vi "saveDelayConfig_烧录.vi"() -> (2 "读取":dbl, 3 "Q写入":dbl, 5 "S写入":dbl)   [LabVIEW 2011]
uses:
  <vilib>/Utility/file.llb/Write To Spreadsheet File (string).vi
  <vilib>/Utility/file.llb/Read From Spreadsheet File (string).vi
panel:
  in  "SFP+写入延时（单位：ms）":dbl
  out "DelayConfigFile":path caption="路径副本"
  in  "保存按钮":bool
  in  "读取延时（单位：ms）":dbl
  in  "QSFP+写入延时（单位：ms）":dbl
  # "建议值：200，可根据实际情况进行调整"
  # "建议值：100，可根据实际情况进行调整"
  # "建议值：100，可根据实际情况进行调整"
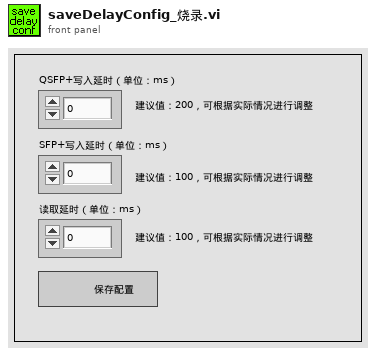
[diagram p1: front panel]
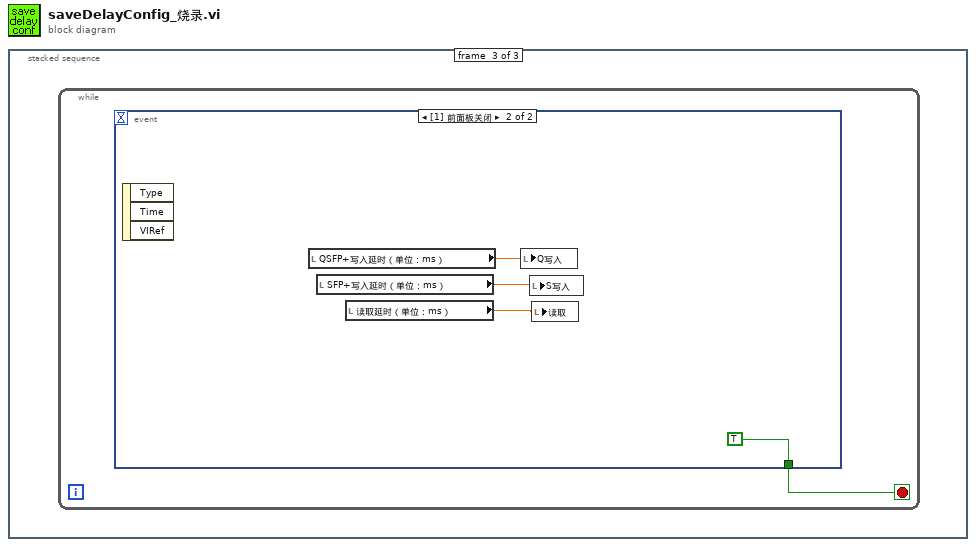
[diagram p0: block diagram]
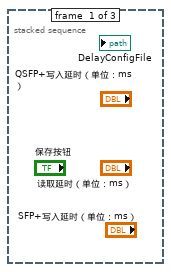
[diagram p2: hidden frame]
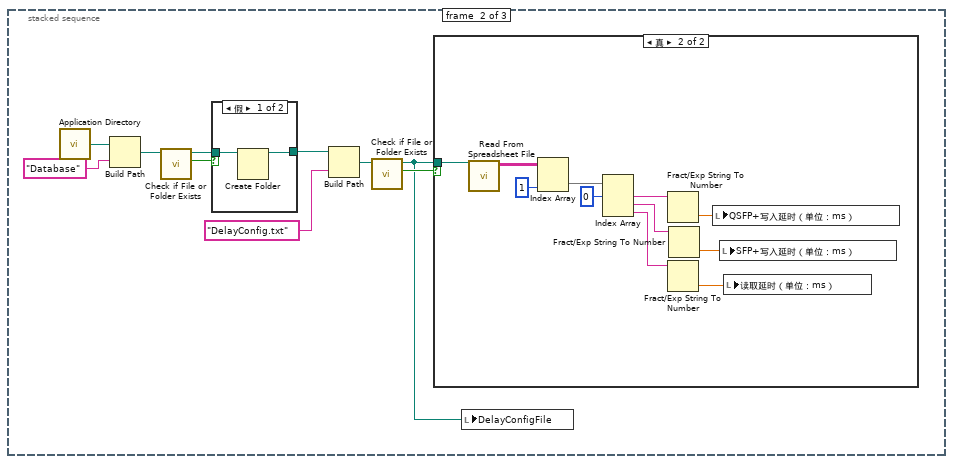
[diagram p3: hidden frame]
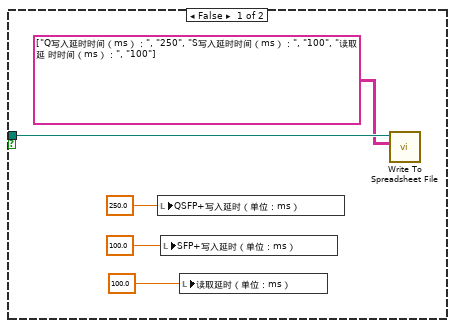
[diagram p4: hidden frame]
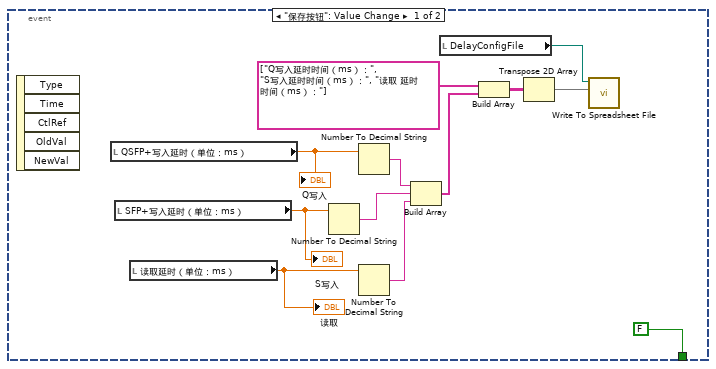
[diagram p6: hidden frame]
diagram:
  n1 = stacked-sequence {
    frame #0 {
    }
    frame #1 {
      n2 = call <vilib>:"Application Directory.vi"() -> ("Application Directory"=w10:path)
      n3 = Build Path(base path=w10, name or relative path="Database" ("名称或相对路径")) -> (appended path=w8:path)
      n4 = call <vilib>:"Check if File or Folder Exists.vi"("path"=w8) -> ("file or folder exists?"=w7:bool, "dup path"=w6:path)  [unwired: 8 in, 1 out]
      n5 = case shown="假" w7 {
        tunnel: w6 -> [w28 w29]
        tunnel: [w27 w29] -> w5
        frame False {
          n6 = Create Folder(path (use dialog)=w28) -> (created path=w27:path)  [unwired: 2 in, 2 out]
        }
        frame True {
        }
      }
      n7 = Build Path(base path=w5, name or relative path="DelayConfig.txt" ("名称或相对路径")) -> (appended path=w3:path)
      n8 = call <vilib>:"Check if File or Folder Exists.vi"("path"=w3) -> ("file or folder exists?"=w2:bool, "dup path"=w1:path)  [unwired: 8 in, 1 out]
      n9 = case shown="真" w2 {
        tunnel: w1 -> [w15 w26]
        frame False {
          n10 = local write "QSFP+写入延时（单位：ms）"(250.0 ("写入延时（单位：ms）")) -> ()
          n11 = local write "SFP+写入延时（单位：ms）"(100.0 ("SFP+写入延时（单位：ms）")) -> ()
          n12 = local write "读取延时（单位：ms）"(100.0 ("读取延时（单位：ms）")) -> ()
          n13 = call-poly <vilib>:"Write To Spreadsheet File.vi"("2D data"=string[][] [["Q写入延时时间（ms）：", "250"], ["S写入延时时间（ms）：", "100"], ["读取 延 时时间（ms）：", "100"]], "file path (dialog if empty)"=w15) -> ()  [unwired: 6 in, 1 out]
        }
        frame True {
          n14 = call-poly <vilib>:"Read From Spreadsheet File.vi"("file path (dialog if empty)"=w26) -> ("all rows"=w25:string[][])  [unwired: 6 in, 4 out]
          n15 = Index Array(array=w25, index (col)=1 ("禁用的索引 (列)")) -> (element=w23:string[])  [unwired: 1 in]
          n16 = Index Array(array=w23, index #1=0 ("索引")) -> (element #1=w21:string, element #2=w16:string, element #3=w18:string)  [unwired: 2 in]
          n17 = Fract/Exp String To Number(string=w21) -> (number=w20:dbl)  [unwired: 3 in, 1 out]
          n18 = Fract/Exp String To Number(string=w18) -> (number=w19:dbl)  [unwired: 3 in, 1 out]
          n19 = Fract/Exp String To Number(string=w16) -> (number=w17:dbl)  [unwired: 3 in, 1 out]
          n20 = local write "QSFP+写入延时（单位：ms）"(w20) -> ()
          n21 = local write "SFP+写入延时（单位：ms）"(w17) -> ()
          n22 = local write "读取延时（单位：ms）"(w19) -> ()
        }
      }
      n23 = local write "DelayConfigFile"(w1) -> ()
    }
    frame #2 {
      n24 = while {
        stop <- w30 stop-if-true
        n25 = event shown="[1] 前面板关闭" {
          selector: _ -> [_ _]
          dyn-events: _ -> [_ _]
          timeout: _ -> [_ _]
          tunnel: [FALSE TRUE] -> w30
          event "保存按钮": Value Change {
            n26 = event-data() -> ()  [unwired: 1 in, 5 out]
            n27 = local read "QSFP+写入延时（单位：ms）"() -> (w42:dbl)
            "Q写入" <- w42
            n28 = local read "SFP+写入延时（单位：ms）"() -> (w31:dbl)
            "S写入" <- w31
            n29 = local read "读取延时（单位：ms）"() -> (w41:dbl)
            "读取" <- w41
            n30 = Number To Decimal String(number=w31) -> (decimal integer string=w33:string)  [unwired: 1 in]
            n31 = Number To Decimal String(number=w42) -> (decimal integer string=w40:string)  [unwired: 1 in]
            n32 = Number To Decimal String(number=w41) -> (decimal integer string=w32:string)  [unwired: 1 in]
            n33 = Build Array(w40, w33, w32) -> (w38:string[])
            n34 = local read "DelayConfigFile"() -> (w34:path)
            n35 = Build Array(string[] ["Q写入延时时间（ms）：", "S写入延时时间（ms）：", "读取 延时 时间（ms）："], w38) -> (w37:string[][])
            n36 = Transpose 2D Array(2D array=w37) -> (transposed array=w35:string[][])
            n37 = call-poly <vilib>:"Write To Spreadsheet File.vi"("2D data"=w35, "file path (dialog if empty)"=w34) -> ()  [unwired: 6 in, 1 out]
          }
          event Panel Close {
            n38 = event-data() -> ()  [unwired: 1 in, 3 out]
            n39 = local read "QSFP+写入延时（单位：ms）"() -> (w43:dbl)
            n40 = local read "SFP+写入延时（单位：ms）"() -> (w44:dbl)
            n41 = local read "读取延时（单位：ms）"() -> (w45:dbl)
            n42 = local write "Q写入"(w43) -> ()
            n43 = local write "S写入"(w44) -> ()
            n44 = local write "读取"(w45) -> ()
          }
        }
      }
    }
  }
